vi "Data_Open(SubVI).vi"(8 "error in (no error)":errorcluster, 11 "DataFilePath":path) -> (0 "error out":errorcluster, 3 "DataArray":dbl[](array[numeric]))   [LabVIEW 2014]
doc: "This SubVI open DataFile and transform data into numeric 1D array"
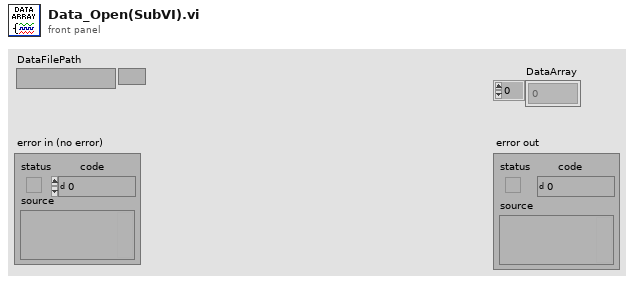
[diagram p1: front panel]
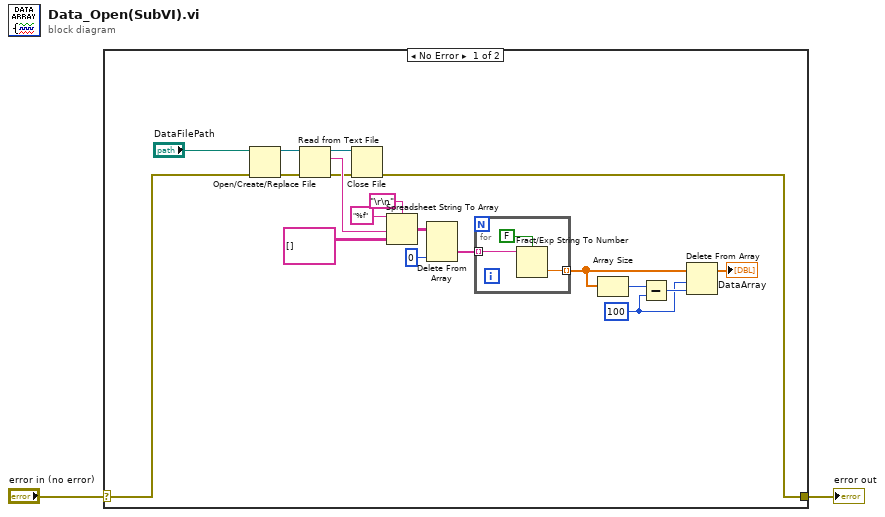
[diagram p0: block diagram]
diagram:
  n1 = case shown="No Error" "error in (no error)" {
    selector: "error in (no error)" -> [w7 w25]
    tunnel: [w6 w25] -> w1
    frame No Error {
      w4 = 100
      n2 = Open/Create/Replace File(file path (use dialog)="DataFilePath", error in=w7) -> (refnum out=w10:refnum<file>, error out=w11:errorcluster)  [unwired: 4 in, 1 out]
      n3 = Read from Text File(file (use dialog)=w10, error in=w11) -> (refnum out=w9:refnum<file>, text=w14:string, error out=w8:errorcluster)  [unwired: 2 in, 1 out]
      n4 = Close File(refnum=w9, error in=w8) -> (error out=w6:errorcluster)  [unwired: 1 out]
      n5 = Spreadsheet String To Array(delimiter (Tab)="\r\n", format string="%f", spreadsheet string=w14, array type (2D Dbl)=string[][] []) -> (array=w16:string[][])
      n6 = Delete From Array(array=w16, index (col)=0 ("disabled index (col)")) -> (deleted portion=w18:string[])  [unwired: 2 in, 1 out]
      n7 = for {
        tunnel: w18 -> [w24] mode=indexing
        tunnel: [w22] -> w19 mode=indexing
        n8 = Fract/Exp String To Number(use system decimal point (T)=FALSE, string=w24) -> (number=w22:dbl)  [unwired: 2 in, 1 out]
      }
      n9 = Array Size(array=w19) -> (size(s)=w20:i32)
      n10 = Subtract(x=w20, y=w4) -> (x-y=w21:i32)
      n11 = Delete From Array(array=w19, length=w4, index=w21) -> (array with subset deleted=→"DataArray":dbl[])  [unwired: 1 out]
    }
    frame Error {
    }
  }
  "error out" <- w1
